vi "IMAQ DLL - Num Not Zero.vi"(0 "IMAQ Ref":T1, 11 "Error In":errorcluster) -> (4 "IMAQ Ref (Dup)":T1, 8 "Non Zero Px Total":u16, 15 "Error Out":errorcluster)   [LabVIEW 2016]
uses:
  <vilib>/vision/Image Controls.llb/IMAQ Image.ctl
  LabView IMAQ Images DLL Files/x64/Release/LabView IMAQ Images.dll
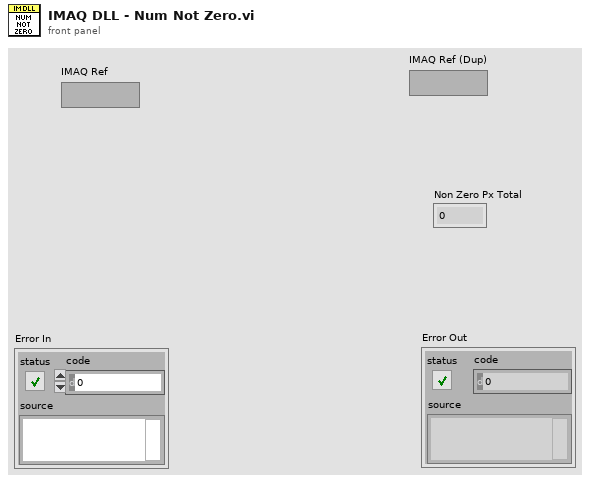
[diagram p1: front panel]
types:
  T1 = typedef "IMAQ Image.ctl" = refnum<image>
  T2 = enum32{"Map Pixel Pointer", "Unmap Pixel Pointer", "Get Pixels Infos"}
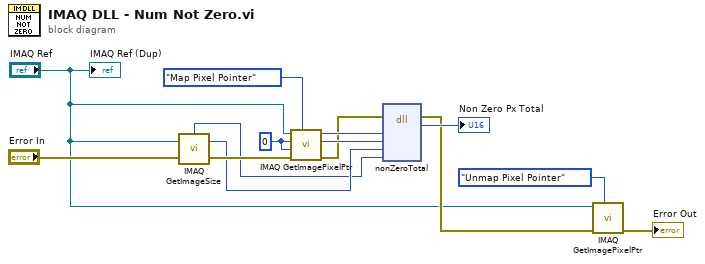
[diagram p0: block diagram]
diagram:
  w12 = 0 ("X Coordinate")
  n1 = call "IMAQ GetImageSize"("Image"="IMAQ Ref", "error in (no error)"="Error In") -> ("Y Resolution"=w10:i32, "X Resolution"=w9:i32, "error out"=w14:errorcluster)  [unwired: 2 in]
  n2 = call "IMAQ GetImagePixelPtr"("Function"=T2."Map Pixel Pointer", "error in (no error)"=w14, "Y Coordinate"=w12, "X Coordinate"=w12, "Image"="IMAQ Ref") -> ("error out"=w8:errorcluster, "LineWidth(Pixels)"=w11:i32, "Pixel Pointer out"=w13:u64)  [unwired: 1 in, 3 out]
  n3 = dll-call lib="D:/Microscope-Control/Tools/LabView IMAQ Images/LabView IMAQ Images DLL Files/x64/Release/LabView IMAQ Images.dll" fn="nonZeroTotal"(error in=w8, "imPointer"=w13, "LV_Line_Width"=w11, "LV_Rows"=w10, "LV_Cols"=w9) -> (error out=w4:errorcluster, "numNotZero"=→"Non Zero Px Total":u16)  [unwired: 6 in, 1 out]
  n4 = call "IMAQ GetImagePixelPtr"("Function"=T2."Unmap Pixel Pointer", "error in (no error)"=w4, "Image"="IMAQ Ref") -> ("error out"=→"Error Out":errorcluster)  [unwired: 3 in, 5 out]
  "IMAQ Ref (Dup)" <- "IMAQ Ref"
